vi "Experiment 2.vi"() -> ()   [LabVIEW 2026]
doc: "Experiment 2"
uses:
  <vilib>/Analysis/baseanly.llb/Mean (DBL).vi
  <vilib>/Analysis/NI_AALBase.lvlib
panel:
  out "Execution Time - Per Call (us)":dbl format="%.6f"
  out "Execution Time - 1M Calls (seconds)":dbl format="%.6f"
  out "Output":dbl[](array[numeric]) format="%.3f"
  # "Experiment 2"
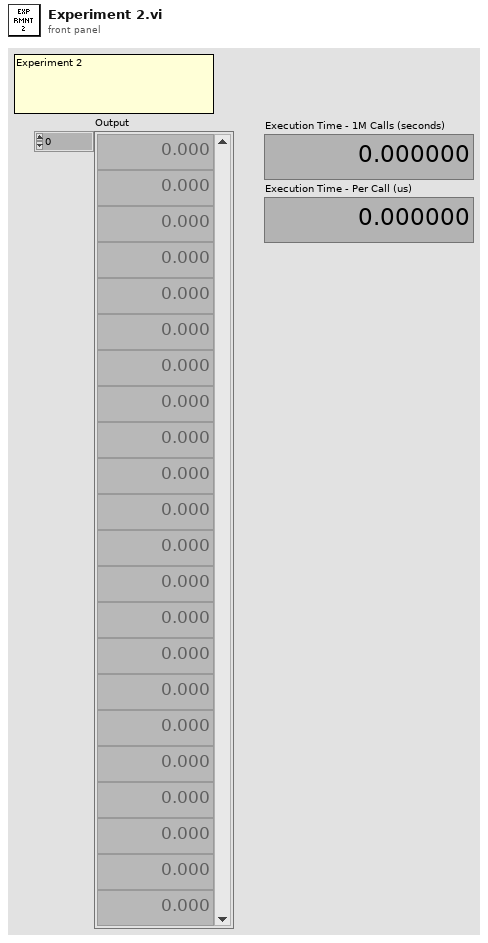
[diagram p1: front panel]
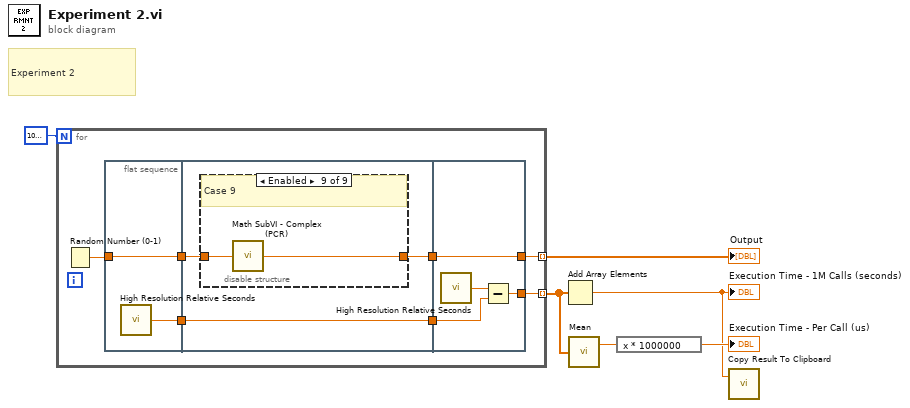
[diagram p0: block diagram]
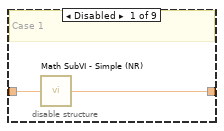
[diagram p2: hidden frame]
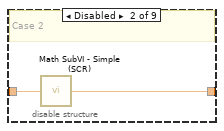
[diagram p3: hidden frame]
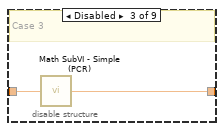
[diagram p4: hidden frame]
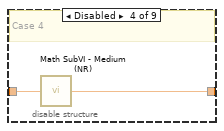
[diagram p5: hidden frame]
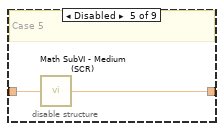
[diagram p6: hidden frame]
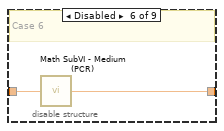
[diagram p7: hidden frame]
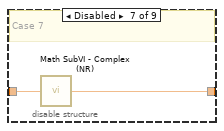
[diagram p8: hidden frame]
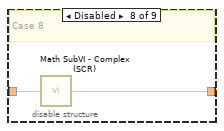
[diagram p9: hidden frame]
diagram:
  # "Experiment 2"
  n1 = for {
    N: 1000000 -> [_]
    tunnel: [w13] -> w6 mode=indexing
    tunnel: [w7] -> w4 mode=indexing
    n2 = Random Number (0-1)() -> (number: 0 to 1=w12:dbl)
    n3 = flat-sequence {
      tunnel: w12 -> [w15]
      tunnel: [w15] -> w11
      tunnel: [w14] -> w8
      tunnel: w11 -> [w16]
      tunnel: [w17] -> w10
      tunnel: [w18] -> w9
      tunnel: w8 -> [w18]
      tunnel: [w40] -> w13
      tunnel: w10 -> [w40]
      tunnel: w9 -> [w38]
      tunnel: [w37] -> w7
      frame #0 {
        n4 = call <vilib>:"High Resolution Relative Seconds.vi"() -> ("relative seconds"=w14:dbl)
      }
      frame #1 {
        n5 = disable-structure shown="Enabled" {
          disable-tunnel: [w20 w22 w24 w26 w28 w30 w32 w34 w36] -> w17
          disable-tunnel: w16 -> [w19 w21 w23 w25 w27 w29 w31 w33 w35]
          frame Disabled {
            # "Case 1"
            n6 = call "Math SubVI - Simple (NR).vi"("Input"=w19) -> ("Output"=w20:dbl)
          }
          frame Disabled {
            # "Case 2"
            n7 = call "Math SubVI - Simple (SCR).vi"("Input"=w21) -> ("Output"=w22:dbl)
          }
          frame Disabled {
            # "Case 3"
            n8 = call "Math SubVI - Simple (PCR).vi"("Input"=w23) -> ("Output"=w24:dbl)
          }
          frame Disabled {
            # "Case 4"
            n9 = call "Math SubVI - Medium (NR).vi"("Input"=w25) -> ("Output"=w26:dbl)
          }
          frame Disabled {
            # "Case 5"
            n10 = call "Math SubVI - Medium (SCR).vi"("Input"=w27) -> ("Output"=w28:dbl)
          }
          frame Disabled {
            # "Case 6"
            n11 = call "Math SubVI - Medium (PCR).vi"("Input"=w29) -> ("Output"=w30:dbl)
          }
          frame Disabled {
            # "Case 7"
            n12 = call "Math SubVI - Complex (NR).vi"("Input"=w31) -> ("Output"=w32:dbl)
          }
          frame Disabled {
            # "Case 8"
            n13 = call "Math SubVI - Complex (SCR).vi"("Input"=w33) -> ("Output"=w34:dbl)
          }
          frame Enabled {
            # "Case 9"
            n14 = call "Math SubVI - Complex (PCR).vi"("Input"=w35) -> ("Output"=w36:dbl)
          }
        }
      }
      frame #2 {
        n15 = call <vilib>:"High Resolution Relative Seconds.vi"() -> ("relative seconds"=w39:dbl)
        n16 = Subtract(x=w39, y=w38) -> (x-y=w37:dbl)
      }
    }
  }
  "Output" <- w6
  n17 = Add Array Elements(numeric array=w4) -> (sum=w1:dbl)
  "Execution Time - 1M Calls (seconds)" <- w1
  n18 = call-poly <vilib>:"Mean.vi"("X"=w4) -> ("mean"=w3:dbl)  [unwired: 1 out]
  n19 = expression code="x * 1000000"(w3) -> (→"Execution Time - Per Call (us)":dbl)
  n20 = call "Copy Result To Clipboard.vi"("Input"=w1) -> ()  [unwired: 1 in]
